vi "frequancy translation for DSBFC (AM).vi"() -> ()   [LabVIEW 2018]
uses:
  <vilib>/express/express analysis/Spectral/Block/exnSpectralBlock spectral measurements RMS poly.vi
  <vilib>/express/express analysis/Spectral/Block/exnSpectralBlock spectral measurements RMS DDT.vi
  <vilib>/express/express analysis/Spectral/XNode/ExpressSpectralMeasurementsBlockNode.xnode
panel:
  out "Waveform Graph 4":dynamicdata(graph)
  out "Waveform Graph 3":dynamicdata(graph)
  out "Waveform Graph 2":dynamicdata(graph)
  in  "stop":bool
  out "Waveform Graph":dynamicdata(graph)
  in  "fc":dbl
  in  "fm":dbl
  in  "ka":dbl
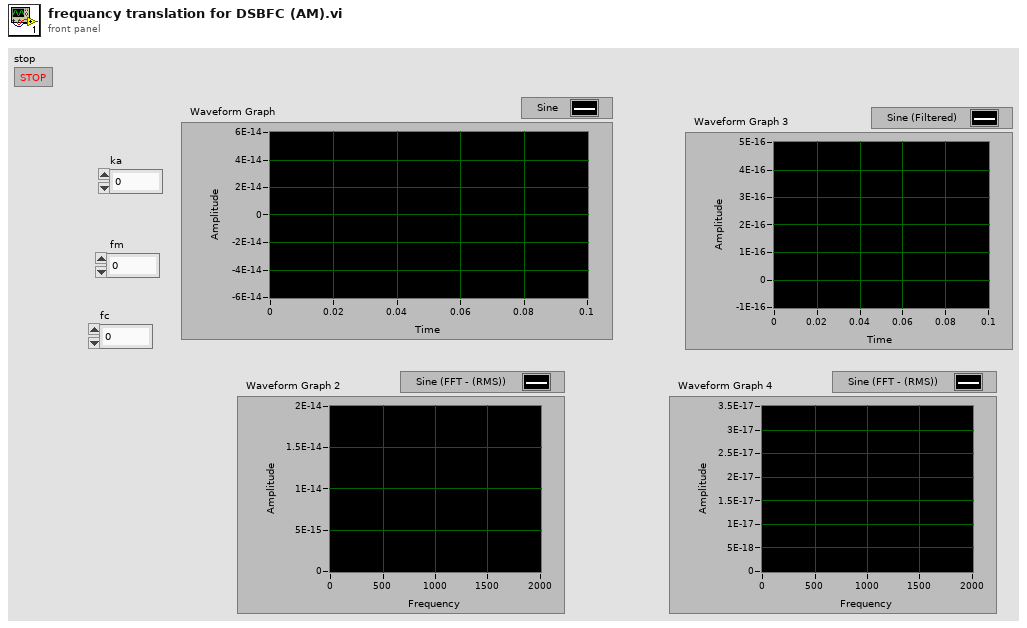
[diagram p1: front panel]
types:
  T1 = cluster{"averaging mode":u16, "weighting mode":u16, "number of averages":u32}
  T2 = cluster{"dB On (F)":bool, "unwrap phase (F)":bool, "convert to degree (F)":bool}
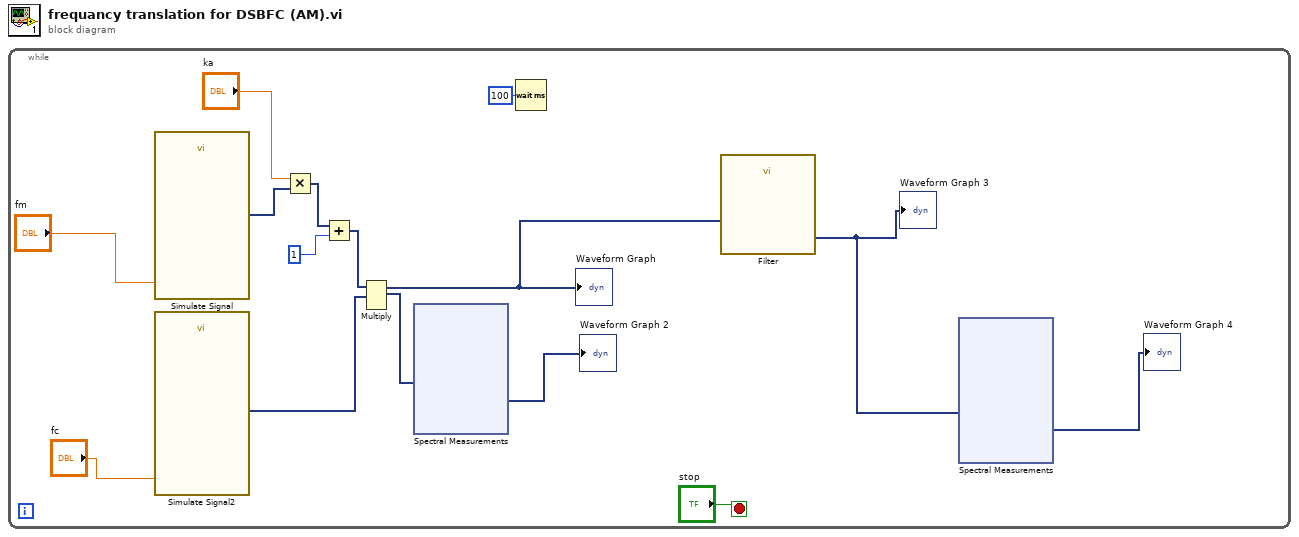
[diagram p0: block diagram]
diagram:
  n1 = while {
    stop <- "stop" stop-if-true
    n2 = call "Simulate Signal"("Frequency"="fm") -> ("Sine"=w11:dynamicdata)  [unwired: 13 in, 1 out]
    n3 = call "Simulate Signal2"("Frequency"="fc") -> ("Sine"=w7:dynamicdata)  [unwired: 13 in, 1 out]
    n4 = Multiply(x="ka", y=w11) -> (x*y=w9:dynamicdata)
    n5 = Add(x=w9, y=1) -> (x+y=w8:dynamicdata)
    n6 = Multiply(1:w7, 2:w8) -> (0:w3:dynamicdata)  [unwired: 1 in, 1 out]
    "Waveform Graph" <- w3
    n7 = xnode "Spectral Measurements"("Signals"=w3) -> ("FFT - (RMS)"=→"Waveform Graph 2":dynamicdata)  [unwired: 1 in, 2 out]
    n8 = Wait (ms)(milliseconds to wait=100) -> ()  [unwired: 1 out]
    n9 = call "Filter"("Signal"=w3) -> ("Filtered Signal"=w1:dynamicdata)  [unwired: 9 in, 1 out]
    "Waveform Graph 3" <- w1
    n10 = xnode "Spectral Measurements"("Signals"=w1) -> ("FFT - (RMS)"=→"Waveform Graph 4":dynamicdata)  [unwired: 1 in, 2 out]
  }
